vi "graph temp and power.vi"(0 "Temperature Graph":refnum<vi>, 7 "T cont":T3 {"utility"."therm volt" format="%_6g"; "utility"."heat volt in" format="%_6g"; "utility"."heat volt out" format="%_6g"; "utility"."power out" format="%_6g"; "utility"."H Vmax" format="%_6g"; "exec"."man power" format="%_6g"; "exec"."exec setpoint" format="%_6g"; "T params"."Settle Time" step=1.0; "T params"."Settle Bandwidth" step=0.01; "T params"."Derivative Tme" step=0.01; "T params"."Integral Time" step=1.0; "T params"."Control Bandwidth" step=0.1; "T params"."Setpoint" step=0.1; "T status"."Setpoint" format="%_6g"; "T status"."Power" format="%_6g"; "T status"."Temp" format="%_6g"}) -> (2 "meas index":i32, 4 "man":bool, 8 "T and P graph":cluster{"t hist":dbl[], "T hist":dbl[]}[](array[cluster]), 15 "T status":T1 {"Setpoint" format="%_6g"; "Power" format="%_6g"; "Temp" format="%_6g"})   [LabVIEW 2019]
doc: "This subVI manages the data extraction for the time, temperature, and power for the full history graph in the bug experiment. It scales the normalized power to the given temperature scale of the graph dynamically.\n\nPaul K Dixon\nP3600\nCSUSB Physics"
uses:
  typedefs/temp cont cluster.ctl
  typedefs/temp exec cluster.ctl
  typedefs/temp mode enum.ctl
  typedefs/temp indicator.ctl
  typedefs/temp control status.ctl
  typedefs/PID control parameters.ctl
  typedefs/temp cont utility.ctl
panel:
  out "P plot":cluster{"t hist":dbl[], dbl[]}
  out "T plot":cluster{"t hist":dbl[], "T hist":dbl[]}
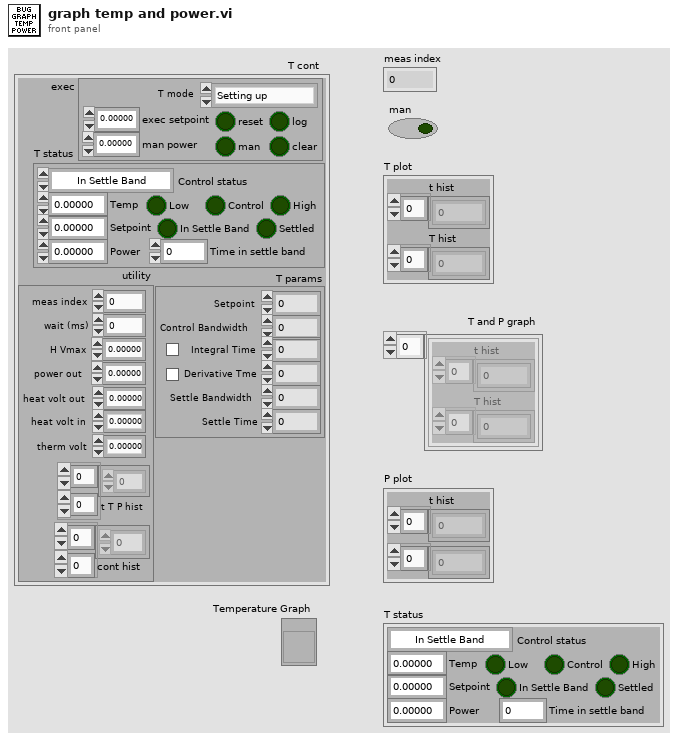
[diagram p1: front panel]
types:
  T1 = typedef "temp indicator.ctl" = cluster{"Control status":T2, "Temp":dbl, "Power":dbl, "Time in settle band":dbl, "Settled":bool, "Low":bool, "High":bool, "Setpoint":dbl, "Control":bool, "In Settle Band":bool}
  T2 = typedef "temp control status.ctl" = enum16{"In Settle Band", "In Control Band", "Below Control Band", "Above Control Band"}
  T3 = typedef "temp cont cluster.ctl" = cluster{"exec":T4, "T status":T1, "T params":T6, "utility":T7}
  T4 = typedef "temp exec cluster.ctl" = cluster{"T mode":T5, "exec setpoint":dbl, "reset":bool, "man power":dbl, "man":bool, "log":bool, "clear":bool}
  T5 = typedef "temp mode enum.ctl" = enum16{"Setting up", "Listening to exec", "Exit"}
  T6 = typedef "PID control parameters.ctl" = cluster{"Setpoint":dbl, "Control Bandwidth":dbl, "Integral Time":dbl, "Int\nON":bool, "Derivative Tme":dbl, "Der\nON":bool, "Settle Bandwidth":dbl, "Settle Time":dbl}
  T7 = typedef "temp cont utility.ctl" = cluster{"meas index":i32, "wait (ms)":i32, "H Vmax":dbl, "power out":dbl, "heat volt out":dbl, "heat volt in":dbl, "therm volt":dbl, "t T P hist":dbl[][], "cont hist":dbl[][]}
  T8 = cluster{"t T P hist":dbl[], "t T P hist":dbl[]}[]
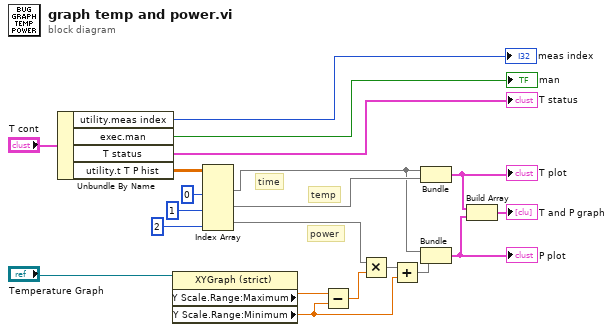
[diagram p0: block diagram]
diagram:
  # "power"
  # "temp"
  # "time"
  n1 = Unbundle By Name("T cont") -> ("utility.meas index"=→"meas index":i32, "exec.man"=→"man":bool, "T status"=→"T status":T1, "utility.t T P hist"=w11:dbl[][])
  n2 = property class="XYGraph (strict)"(reference="Temperature Graph") -> ("Y Scale.Range:Maximum"=w17:dbl, "Y Scale.Range:Minimum"=w16:dbl)  [unwired: 1 in, 2 out]
  n3 = Index Array(array=w11, index (col) #1=0 ("disabled index (col)"), index (col) #2=1 ("index (col)"), index (col) #3=2 ("index (col)")) -> (element #1=w8:dbl[], element #2=w10:dbl[], element #3=w9:dbl[])  [unwired: 3 in]
  n4 = Subtract(x=w17, y=w16) -> (x-y=w14:dbl)
  n5 = Multiply(x=w9, y=w14) -> (x*y=w15:dbl[])
  n6 = Add(x=w15, y=w16) -> (x+y=w13:dbl[])
  n7 = Bundle("t T P hist"=w8, "t T P hist"=w10) -> (w6:cluster{"t T P hist":dbl[], "t T P hist":dbl[]})  [unwired: 1 in]
  "T plot" <- w6
  n8 = Bundle("t T P hist"=w8, w13) -> (w5:cluster{"t T P hist":dbl[], dbl[]})  [unwired: 1 in]
  "P plot" <- w5
  n9 = Build Array(w6, w5) -> (→"T and P graph":T8)
